vi "更新报警信息.vi"(11 "添加的数组":refnum<vi>[](array[refnum])) -> ()   [LabVIEW 2017]
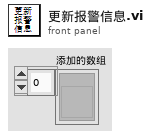
[diagram p1: front panel]
types:
  T1 = typedef "Component Assemble Input.ctl" = cluster{"Component Name":string, "Component State":bool, "D Value":i32}
  T2 = typedef "MX操作选项.ctl" = enum16{"MX Initial ", "MX Close", "X&Y&M Read", "X&Y&M Write", "D Read", "D Write", "Many component Read", "Many component Write", "Load Function Global"}
  T3 = cluster{"%Y_%m_%d_%H_%M_%S%3u":string, "%Y_%m_%d":string, "%H_%M_%S%3u":string}
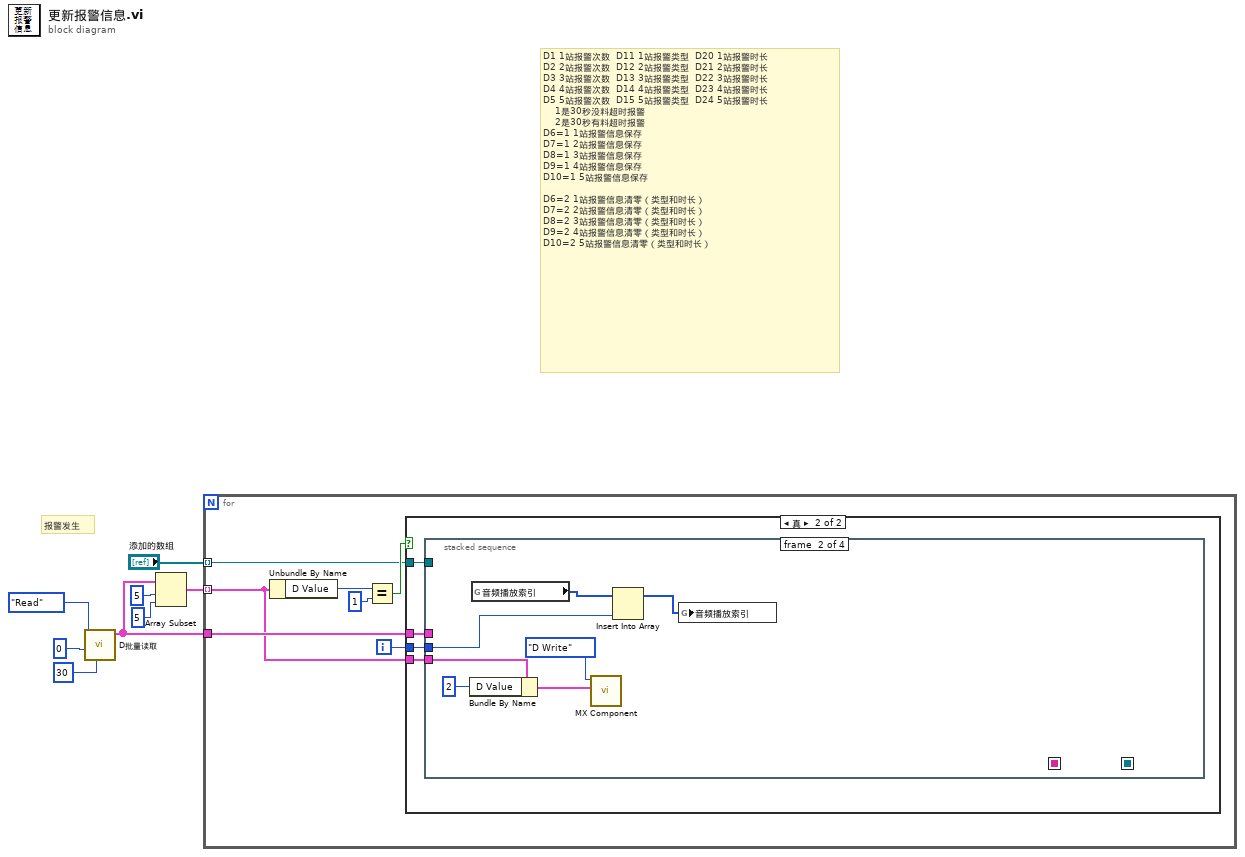
[diagram p0: block diagram]
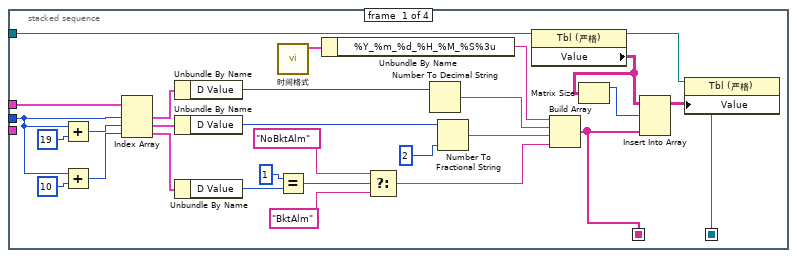
[diagram p3: hidden frame]
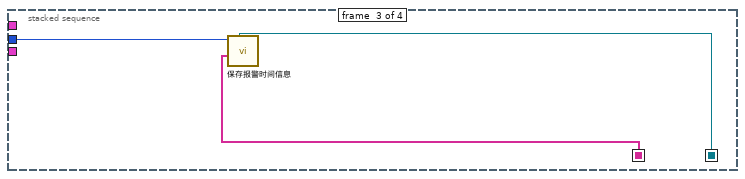
[diagram p4: hidden frame]
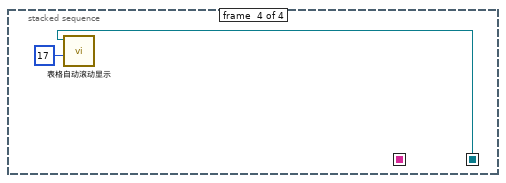
[diagram p5: hidden frame]
diagram:
  # "D1\t1站报警次数\t\tD11\t1站报警类型\t\tD20\t1站报警时长\nD2\t2站报警次数\t\tD12\t2站报警类型\t\tD21\t2站报警时长\nD3\t3站报警次数\t\tD13\t3站报警类型\t\tD22\t3站报警时长\nD4\t4站报警次数\t\tD14\t4站报警类型\t\tD23\t4站报警时长\nD5\t5站报警次数\t\tD15\t5站报警类型\t\tD24\t5站报警时长\n\t\t\t\t1是30秒没料超时报警\t\t\t\n\t\t\t\t2是30秒有料超时报警\t\t\t\nD6=1\t1站报警信息保存\t\t\t\t\t\t\nD7=1\t2站报警信息保存\t\t\t\t\t\t\nD8=1\t3站报警信息保存\t\t\t\t\t\t\nD9=1\t4站报警信息保存\t\t\t\t\t\t\nD10=1\t5站报警信息保存\t\t\t\t\t\t\n\t\t\t\t\t\t\t\nD6=2\t1站报警信息清零（类型和时长）\t\t\t\t\t\t\nD7=2\t2站报警信息清零（类型和时长）\t\t\t\t\t\t\nD8=2\t3站报警信息清零（类型和时长）\t\t\t\t\t\t\nD9=2\t4站报警信息清零（类型和时长）\t\t\t\t\t\t\nD10=2\t5站报警信息清零（类型和时长）"
  # "报警发生"
  n1 = call "D批量读取.vi"("长度"=30 ("数值"), "开始"=0, "选项"=enum16{"Read", "Write"}."Read") -> ("D读取"=w4:T1[])  [unwired: 7 in, 1 out]
  n2 = Array Subset(array=w4, index=5 ("索引"), length=5 ("长度")) -> (w5:T1[])
  n3 = for {
    tunnel: w5 -> [w9] mode=indexing
    tunnel: w4 -> [w12]
    tunnel: "添加的数组" -> [w10] mode=indexing
    i -> [w11]
    n4 = Unbundle By Name(w9) -> ("D Value"=w15:i32)
    n5 = Equal?(x=w15, y=1) -> (x = y?=w13:bool)
    n6 = case shown="真" w13 {
      tunnel: w12 -> [_ w19]
      tunnel: w11 -> [_ w18]
      tunnel: w10 -> [_ w17]
      tunnel: w9 -> [_ w16]
      frame False {
      }
      frame True {
        n7 = stacked-sequence {
          seq-local: [w23 _ _ _] -> [_ _ w57 _]
          seq-local: [w22 _ _ _] -> [_ _ w56 w59]
          tunnel: w19 -> [w48 _ _ _]
          tunnel: w18 -> [w45 w50 w58 _]
          tunnel: w17 -> [w31 _ _ _]
          tunnel: w16 -> [_ w54 _ _]
          frame #0 {
            n8 = Add(x=w45, y=19) -> (x+y=w46:i32)
            n9 = Add(x=w45, y=10) -> (x+y=w43:i32)
            n10 = Index Array(array=w48, index #1=w45, index #2=w46, index #3=w43) -> (element #1=w40:T1, element #2=w39:T1, element #3=w38:T1)
            n11 = Unbundle By Name(w40) -> ("D Value"=w37:i32)
            n12 = Unbundle By Name(w39) -> ("D Value"=w34:i32)
            n13 = Unbundle By Name(w38) -> ("D Value"=w35:i32)
            n14 = call "时间格式.vi"() -> ("时间格式"=w42:T3)  [unwired: 11 in]
            n15 = Equal?(x=1, y=w35) -> (x = y?=w28:bool)
            n16 = Unbundle By Name(w42) -> ("%Y_%m_%d_%H_%M_%S%3u"=w41:string)
            n17 = Select(t="NoBktAlm", s=w28, f="BktAlm") -> (s? t:f=w26:string)
            n18 = Number To Decimal String(number=w37) -> (decimal integer string=w36:string)  [unwired: 1 in]
            n19 = Number To Fractional String(number=w34, precision (6)=i16 2 ("精度(6)")) -> (F-format string=w33:string)  [unwired: 2 in]
            n20 = property class="Tbl (严格)"(reference=w31) -> (reference out=w29:refnum<vi>, "Value"=w21:string[][])  [unwired: 1 in, 1 out]
            n21 = Build Array(w41, w36, w33, w26) -> (w23:string[])
            n22 = Matrix Size(0:w21) -> (1:w20:i32)  [unwired: 1 out]
            n23 = Insert Into Array(array=w21, index (row)=w20, new element=w23) -> (w30:string[][])  [unwired: 1 in]
            n24 = property class="Tbl (严格)"(reference=w29, "Value"=w30) -> (reference out=w22:refnum<vi>)  [unwired: 1 in, 1 out]
          }
          frame #1 {
            n25 = Bundle By Name(cluster=w54, "D Value"=2) -> (w52:T1)
            n26 = global read "全局 1.vi" "音频播放索引"() -> (w51:i32[])
            n27 = call "MX Component.vi"("Component Assemble Input"=w52, "MX操作选项"=MX操作选项."D Write") -> ()  [unwired: 7 in, 3 out]
            n28 = Insert Into Array(array=w51, new element=w50) -> (w49:i32[])  [unwired: 1 in]
            n29 = global write "全局 1.vi" "音频播放索引"(w49) -> ()
          }
          frame #2 {
            n30 = call "保存报警时间信息.vi"("表格 5"=w56, "InsertData"=w57, "设备编号"=w58) -> ()  [unwired: 9 in]
          }
          frame #3 {
            n31 = call "表格自动滚动显示.vi"("显示行数"=u32 17, "表格控件"=w59) -> ()  [unwired: 10 in]
          }
        }
      }
    }
  }
